vi "Stop Move piezo.vi"(8 "error in (no error)":errorcluster, 9 "notifier out":refnum<notifier>, 10 "MOVE TO [MICRON]":dbl=1.0 format="%0.2f", 11 "Hardware Configuration in":T1) -> (0 "error out":errorcluster, 3 "Hardware Configuration out":T1)   [LabVIEW 2013, in "Piezo.lvlib"]
uses:
  Piezo/Piezo.lvlib
  Hardware Configuration Piezo.ctl
  Piezo/Piezo display.ctl
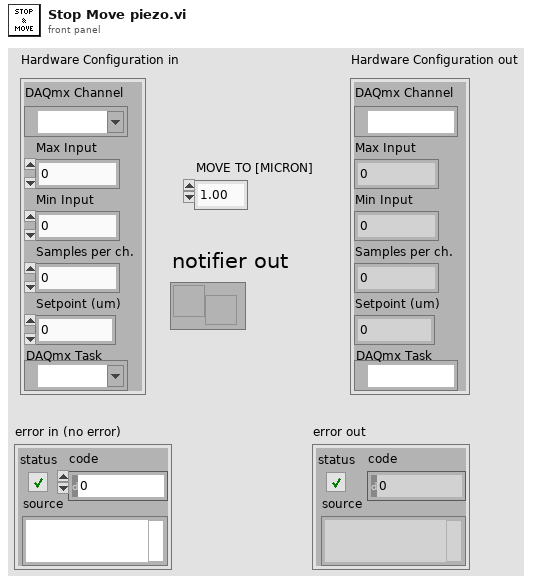
[diagram p1: front panel]
types:
  T1 = typedef "Piezo.lvlib/Hardware Configuration Piezo.ctl" = cluster{"DAQmx Channel":tag, "Max Input":dbl, "Min Input":dbl, "Samples per ch.":dbl, "Setpoint (um)":dbl, "DAQmx Task":refnum<k21>}
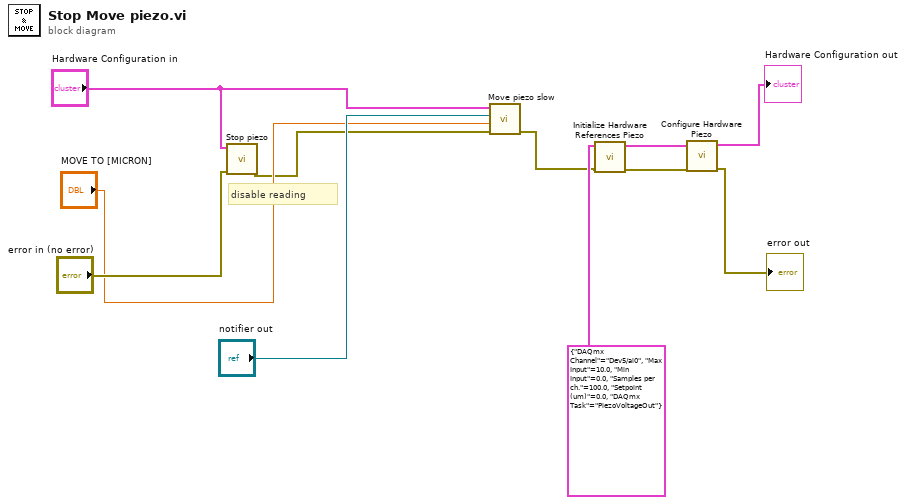
[diagram p0: block diagram]
diagram:
  # "disable reading"
  n1 = call "Stop piezo.vi"("error in (no error)"="error in (no error)", "Hardware Configuration"="Hardware Configuration in") -> ("error out"=w2:errorcluster)  [unwired: 9 in]
  n2 = call "Move piezo slow.vi"("error in (no error)"=w2, "MOVE TO [MICRON]"="MOVE TO [MICRON]", "notifier out"="notifier out", "Hardware Configuration"="Hardware Configuration in") -> ("error out"=w1:errorcluster)  [unwired: 5 in, 1 out]
  n3 = call "Initialize Hardware References Piezo.vi"("error in (no error)"=w1, "Hardware Configuration"=T1 {"DAQmx Channel"="Dev5/ai0", "Max Input"=10.0, "Min Input"=0.0, "Samples per ch."=100.0, "Setpoint (um)"=0.0, "DAQmx Task"="PiezoVoltageOut"}) -> ("error out"=w10:errorcluster, "Hardware Configuration 2"=w11:T1)  [unwired: 8 in]
  n4 = call "Configure Hardware Piezo.vi"("error in (no error)"=w10, "Hardware Configuration in"=w11) -> ("error out"=→"error out":errorcluster, "Hardware Configuration out"=→"Hardware Configuration out":T1)  [unwired: 8 in]
